vi "PinMapService GetPinMap.vi"(6 "contextId":T1, 8 "error in":errorcluster, 9 "timeout (ms)":i32=-1, 10 "Request Data":T3, 11 "gRPC ID":T1) -> (0 "error out":errorcluster, 2 "Response Data":T2, 3 "gRPC ID out":T1)   [LabVIEW 2020, in "ni.measurementlink.pinmap.v1.lvlib"]
uses:
  ni.measurementlink.pinmap.v1.lvlib
  14035477-4c25-4107-8ed5-d0c4ef420ce5.vi
  RPC Messages/ni_measurementlink_pinmap_v1_PinMap_Flat.ctl
  <vilib>/gRPC/LabVIEW gRPC Library/Shared/grpcId.ctl
  <vilib>/gRPC/LabVIEW gRPC Library/grpc-lvsupport-release.lvlib
  RPC Messages/ni_measurementlink_pinmap_v1_PinMap.ctl
  RPC Messages/ni_measurementlink_pinmap_v1_GetPinMapRequest.ctl
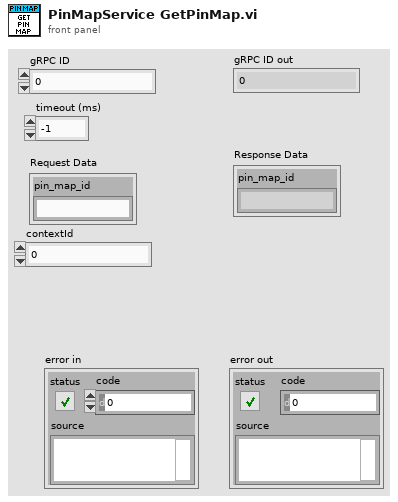
[diagram p1: front panel]
types:
  T1 = typedef "grpc-lvsupport-release.lvlib/grpcId.ctl" = u64
  T2 = typedef "ni.measurementlink.pinmap.v1.lvlib/ni_measurementlink_pinmap_v1_PinMap.ctl" = cluster{"pin_map_id":string}
  T3 = typedef "ni.measurementlink.pinmap.v1.lvlib/ni_measurementlink_pinmap_v1_GetPinMapRequest.ctl" = cluster{"pin_map_id":string}
  T4 = typedef "ni.measurementlink.pinmap.v1.lvlib/ni_measurementlink_pinmap_v1_PinMap_Flat.ctl" = cluster{"pin_map_id":string}
  T5 = typedef "ni.measurementlink.pinmap.v1.lvlib/ni_measurementlink_pinmap_v1_GetPinMapRequest_Flat.ctl" = cluster{"pin_map_id":string}
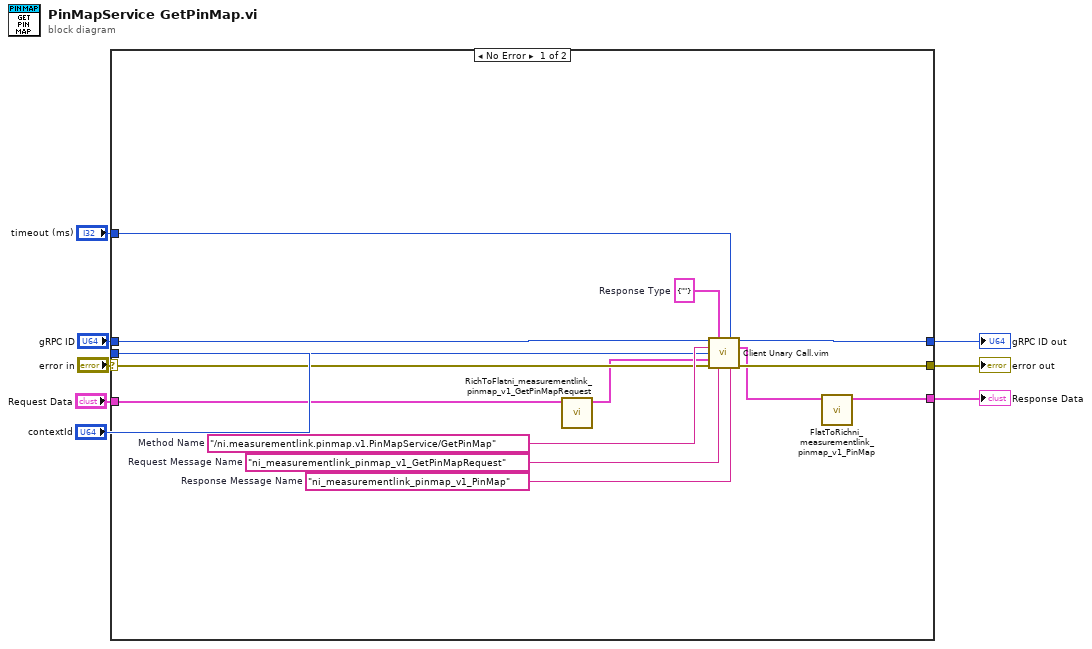
[diagram p0: block diagram]
diagram:
  n1 = case shown="No Error" "error in" {
    selector: "error in" -> [w18 w23]
    tunnel: [w17 w23] -> w7
    tunnel: "gRPC ID" -> [w16 w24]
    tunnel: [w15 w24] -> w5
    tunnel: "Request Data" -> [w12 _]
    tunnel: [w9 _] -> w3
    tunnel: "timeout (ms)" -> [w14 _]
    tunnel: "contextId" -> [w13 _]
    frame No Error {
      w19 = "ni_measurementlink_pinmap_v1_PinMap"  # Response Message Name
      w20 = "ni_measurementlink_pinmap_v1_GetPinMapRequest"  # Request Message Name
      w21 = T4 {"pin_map_id"=""}  # Response Type
      w22 = "/ni.measurementlink.pinmap.v1.PinMapService/GetPinMap"  # Method Name
      n2 = call "RichToFlatni_measurementlink_pinmap_v1_GetPinMapRequest.vi"("InputCluster"=w12) -> ("OutputCluster"=w11:T5)  [unwired: 10 in]
      n3 = call "Client Unary Call.vim"("ClientID in"=w16, "Response Type"=w21, "timeout (ms)"=w14, "Method Name"=w22, "contextId"=w13, "Request Data"=w11, "error in"=w18, "Request Message Name"=w20, "Response Message Name"=w19) -> ("ClientID out"=w15:u64, "Response Data"=w10:T4, "error out"=w17:errorcluster)  [unwired: 4 in]
      n4 = call "FlatToRichni_measurementlink_pinmap_v1_PinMap.vi"("InputCluster"=w10) -> ("OutputCluster"=w9:T2)  [unwired: 10 in]
    }
    frame Error {
    }
  }
  "error out" <- w7
  "gRPC ID out" <- w5
  "Response Data" <- w3
